vi "TestExec.Data to RetDataStr.vi"(3 "error in":errorcluster, 5 "Data":variant) -> (0 "error out":errorcluster, 2 "RetStr":string)   [LabVIEW 2017]
uses:
  <vilib>/Utility/Data Type/NI_Data Type.lvlib
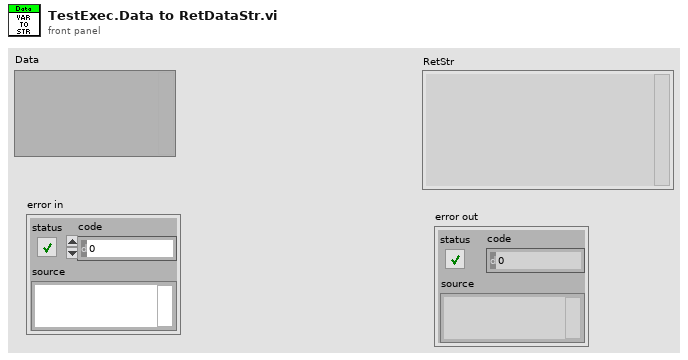
[diagram p1: front panel]
types:
  T1 = typedef "NI_Data Type.lvlib/Data Type.ctl" = enum8{"Invalid Type", "Void", "I8", "I16", "I32", "I64", "U8", "U16", "U32", "U64", "Single Float", "Double Float", "Extended Float", "Single Complex", "Double Complex", "Extended Complex", "Enum U8", "Enum U16", "Enum U32", "Enum U64", "Single Float With Unit", "Double Float With Unit", "Extended Float With Unit", "Single Complex with Unit", "Double Complex with Unit", "Extended Complex with Unit", "Boolean", "String", "Path", "Picture", "Tag", "Array", "Cluster", "Variant", "LV Variant", "Waveform", "Timestamp", "Digital Waveform", "Digital Data", "ExpressData", "Refnum", "External Data", "VI", "Poly VI", "LabVIEW Class Instance", "Fixed Point"}
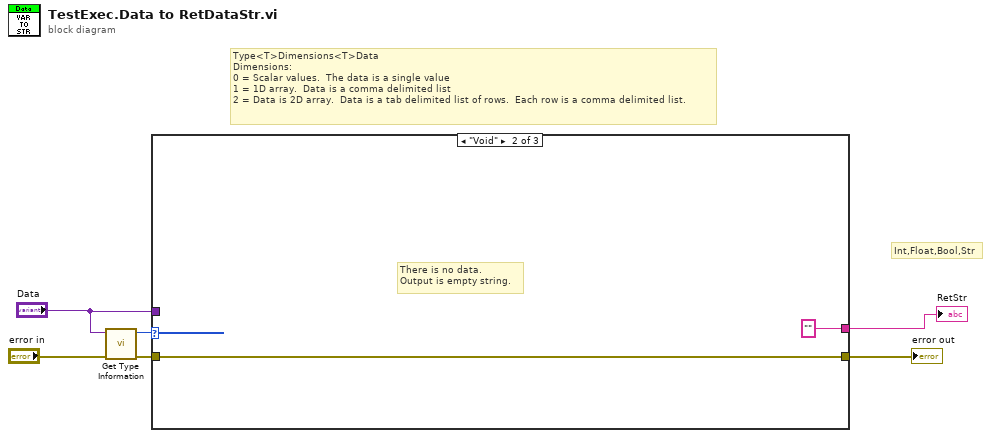
[diagram p0: block diagram]
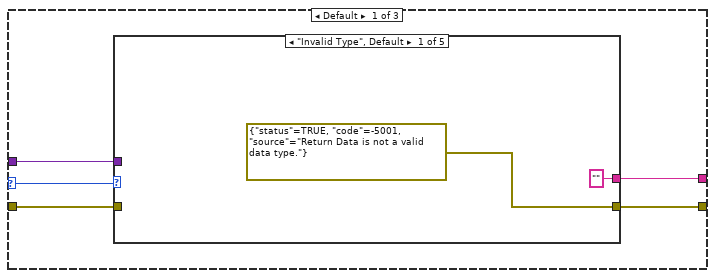
[diagram p2: hidden frame]
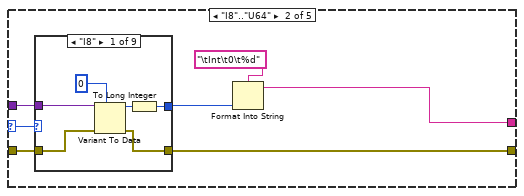
[diagram p3: hidden frame]
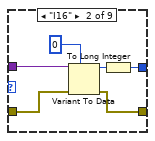
[diagram p4: hidden frame]
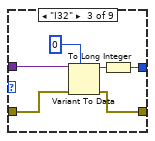
[diagram p5: hidden frame]
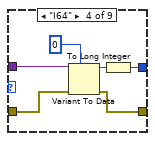
[diagram p6: hidden frame]
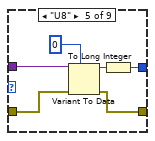
[diagram p7: hidden frame]
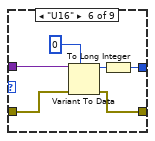
[diagram p8: hidden frame]
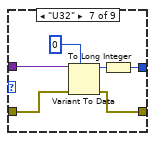
[diagram p9: hidden frame]
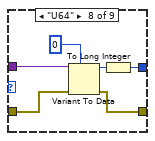
[diagram p10: hidden frame]
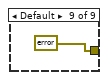
[diagram p11: hidden frame]
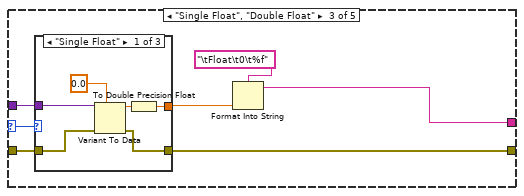
[diagram p12: hidden frame]
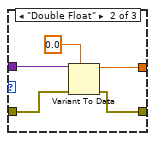
[diagram p13: hidden frame]
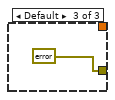
[diagram p14: hidden frame]
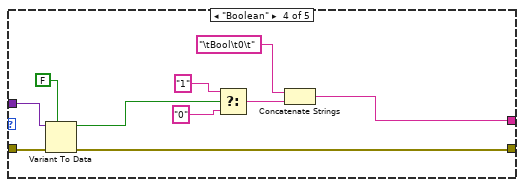
[diagram p15: hidden frame]
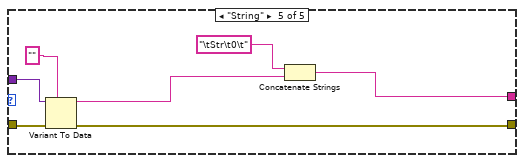
[diagram p16: hidden frame]
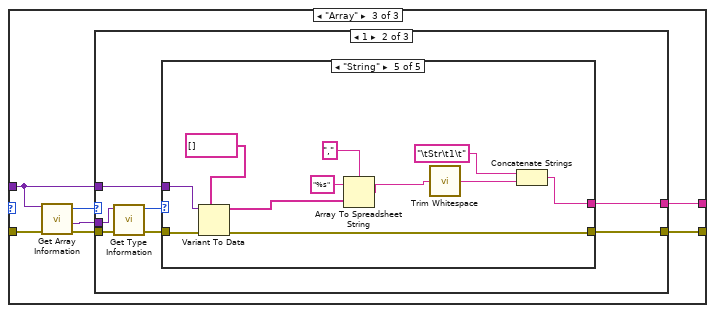
[diagram p17: hidden frame]
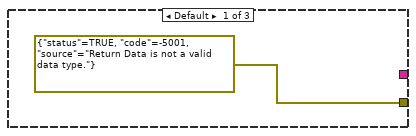
[diagram p18: hidden frame]
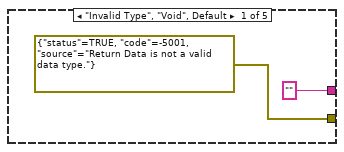
[diagram p19: hidden frame]
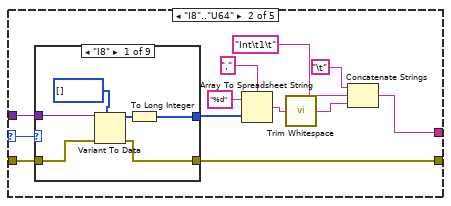
[diagram p20: hidden frame]
diagram:
  # "Type<T>Dimensions<T>Data\nDimensions:\n0 = Scalar values.  The data is a single value\n1 = 1D array.  Data is a comma delimited list\n2 = Data is 2D array.  Data is a tab delimited list of rows.  Each row is a comma delimited list."
  # "Int,Float,Bool,Str"
  n1 = call <vilib>:"Get Type Information.vi"("error in (no error)"="error in", "Variant"="Data") -> ("error out"=w5:errorcluster, "Type"=w3:T1)  [unwired: 5 in, 3 out]
  n2 = case shown="\"Void\"" w3 {
    selector: w3 -> [w7 _ _]
    tunnel: w5 -> [w11 w106 w112]
    tunnel: "Data" -> [w10 _ w111]
    tunnel: [w9 "" w114] -> w1
    tunnel: [w8 w106 w113] -> w4
    frame Default {
      n3 = case shown="\"Invalid Type\", Default" w7 {
        selector: w7 -> [_ w19 w75 _ _]
        tunnel: w11 -> [_ w18 w74 w98 w105]
        tunnel: [errorcluster {"status"=TRUE, "code"=-5001, "source"="Return Data is not a valid data type."} ("error constant") w15 w71 w89 w101] -> w8
        tunnel: ["" w16 w72 w90 w102] -> w9
        tunnel: w10 -> [_ w20 w76 w97 w104]
        frame "Invalid Type", Default {
        }
        frame "I8".."U64" {
          n4 = case shown="\"I8\"" w19 {
            tunnel: w20 -> [w26 w32 w38 w44 w50 w56 w62 w68 _]
            tunnel: [w23 w29 w35 w41 w47 w53 w59 w65 _] -> w17
            tunnel: w18 -> [w22 w28 w34 w40 w46 w52 w58 w64 _]
            tunnel: [w21 w27 w33 w39 w45 w51 w57 w63 errorcluster {"status"=TRUE, "code"=-5001, "source"="Return Data is not a valid data type."} ("error constant")] -> w15
            frame "I8" {
              n5 = Variant To Data(error in=w22, type=i8 0, Variant=w26) -> (data=w24:i8, error out=w21:errorcluster)
              n6 = To Long Integer(number=w24) -> (32bit integer=w23:i32)
            }
            frame "I16" {
              n7 = Variant To Data(error in=w28, type=i16 0, Variant=w32) -> (data=w30:i16, error out=w27:errorcluster)
              n8 = To Long Integer(number=w30) -> (32bit integer=w29:i32)
            }
            frame "I32" {
              n9 = Variant To Data(error in=w34, type=0, Variant=w38) -> (data=w36:i32, error out=w33:errorcluster)
              n10 = To Long Integer(number=w36) -> (32bit integer=w35:i32)
            }
            frame "I64" {
              n11 = Variant To Data(error in=w40, type=i64 0, Variant=w44) -> (data=w42:i64, error out=w39:errorcluster)
              n12 = To Long Integer(number=w42) -> (32bit integer=w41:i32)
            }
            frame "U8" {
              n13 = Variant To Data(error in=w46, type=u8 0, Variant=w50) -> (data=w48:u8, error out=w45:errorcluster)
              n14 = To Long Integer(number=w48) -> (32bit integer=w47:i32)
            }
            frame "U16" {
              n15 = Variant To Data(error in=w52, type=u16 0, Variant=w56) -> (data=w54:u16, error out=w51:errorcluster)
              n16 = To Long Integer(number=w54) -> (32bit integer=w53:i32)
            }
            frame "U32" {
              n17 = Variant To Data(error in=w58, type=u32 0, Variant=w62) -> (data=w60:u32, error out=w57:errorcluster)
              n18 = To Long Integer(number=w60) -> (32bit integer=w59:i32)
            }
            frame "U64" {
              n19 = Variant To Data(error in=w64, type=u64 0, Variant=w68) -> (data=w66:u64, error out=w63:errorcluster)
              n20 = To Long Integer(number=w66) -> (32bit integer=w65:i32)
            }
            frame Default {
            }
          }
          n21 = Format Into String(format string="\tInt\t0\t%d", w17) -> (resulting string=w16:string)  [unwired: 2 in, 1 out]
        }
        frame "Single Float", "Double Float" {
          n22 = case shown="\"Single Float\"" w75 {
            tunnel: w76 -> [w82 w87 _]
            tunnel: [w79 w83 _] -> w73
            tunnel: w74 -> [w78 w85 _]
            tunnel: [w77 w84 errorcluster {"status"=TRUE, "code"=-5001, "source"="Return Data is not a valid data type."} ("error constant")] -> w71
            frame "Single Float" {
              n23 = Variant To Data(error in=w78, type=sgl 0.0, Variant=w82) -> (data=w80:sgl, error out=w77:errorcluster)
              n24 = To Double Precision Float(number=w80) -> (double precision float=w79:dbl)
            }
            frame "Double Float" {
              n25 = Variant To Data(error in=w85, type=0.0, Variant=w87) -> (data=w83:dbl, error out=w84:errorcluster)
            }
            frame Default {
            }
          }
          n26 = Format Into String(format string="\tFloat\t0\t%f", w73) -> (resulting string=w72:string)  [unwired: 2 in, 1 out]
        }
        frame "Boolean" {
          n27 = Variant To Data(error in=w98, type=FALSE, Variant=w97) -> (data=w95:bool, error out=w89:errorcluster)
          n28 = Select(t="1", s=w95, f="0") -> (s? t:f=w94:string)
          n29 = Concatenate Strings("\tBool\t0\t", w94) -> (w90:string)
        }
        frame "String" {
          n30 = Variant To Data(error in=w105, type="", Variant=w104) -> (data=w99:string, error out=w101:errorcluster)
          n31 = Concatenate Strings("\tStr\t0\t", w99) -> (w102:string)
        }
      }
    }
    frame "Void" {
      # "There is no data.\nOutput is empty string."
    }
    frame "Array" {
      n32 = call <vilib>:"Get Array Information.vi"("error in (no error)"=w112, "Variant"=w111) -> ("error out"=w110:errorcluster, "Array Element Data Type"=w108:variant, "Number of Dimensions"=w109:i32)  [unwired: 6 in, 1 out]
      n33 = case shown="1" w109 {
        tunnel: [_ w122 w239] -> w114
        tunnel: [errorcluster {"status"=TRUE, "code"=-5001, "source"="Return Data is not a valid data type."} ("error constant") w121 w238] -> w113
        tunnel: w111 -> [_ w120 w237]
        tunnel: w110 -> [_ w119 w236]
        tunnel: w108 -> [_ w118 w235]
        frame Default {
        }
        frame 1 {
          n34 = call <vilib>:"Get Type Information.vi"("error in (no error)"=w119, "Variant"=w118) -> ("error out"=w116:errorcluster, "Type"=w117:T1)  [unwired: 5 in, 3 out]
          n35 = case shown="\"String\"" w117 {
            selector: w117 -> [_ w135 w195 _ _]
            tunnel: w116 -> [_ w134 w194 w221 w232]
            tunnel: [errorcluster {"status"=TRUE, "code"=-5001, "source"="Return Data is not a valid data type."} ("error constant") w133 w193 w217 w228] -> w121
            tunnel: ["" w128 w188 w218 w229] -> w122
            tunnel: w120 -> [_ w136 w196 w220 w231]
            frame "Invalid Type", "Void", Default {
            }
            frame "I8".."U64" {
              n36 = case shown="\"I8\"" w135 {
                tunnel: w136 -> [w142 w148 w153 w159 w165 w171 w177 w183 _]
                tunnel: [w140 w146 w149 w157 w163 w169 w175 w181 _] -> w132
                tunnel: w134 -> [w139 w145 w152 w156 w162 w168 w174 w180 _]
                tunnel: [w138 w144 w151 w155 w161 w167 w173 w179 errorcluster {"status"=TRUE, "code"=-5001, "source"="Return Data is not a valid data type."} ("error constant")] -> w133
                frame "I8" {
                  n37 = Variant To Data(error in=w139, type=i8[] [], Variant=w142) -> (data=w141:i8[], error out=w138:errorcluster)
                  n38 = To Long Integer(number=w141) -> (32bit integer=w140:i32[])
                }
                frame "I16" {
                  n39 = Variant To Data(error in=w145, type=i16[] [], Variant=w148) -> (data=w147:i16[], error out=w144:errorcluster)
                  n40 = To Long Integer(number=w147) -> (32bit integer=w146:i32[])
                }
                frame "I32" {
                  n41 = Variant To Data(error in=w152, type=i32[] [], Variant=w153) -> (data=w149:i32[], error out=w151:errorcluster)
                }
                frame "I64" {
                  n42 = Variant To Data(error in=w156, type=i64[] [], Variant=w159) -> (data=w158:i64[], error out=w155:errorcluster)
                  n43 = To Long Integer(number=w158) -> (32bit integer=w157:i32[])
                }
                frame "U8" {
                  n44 = Variant To Data(error in=w162, type=u8[] [], Variant=w165) -> (data=w164:u8[], error out=w161:errorcluster)
                  n45 = To Long Integer(number=w164) -> (32bit integer=w163:i32[])
                }
                frame "U16" {
                  n46 = Variant To Data(error in=w168, type=u16[] [], Variant=w171) -> (data=w170:u16[], error out=w167:errorcluster)
                  n47 = To Long Integer(number=w170) -> (32bit integer=w169:i32[])
                }
                frame "U32" {
                  n48 = Variant To Data(error in=w174, type=u32[] [], Variant=w177) -> (data=w176:u32[], error out=w173:errorcluster)
                  n49 = To Long Integer(number=w176) -> (32bit integer=w175:i32[])
                }
                frame "U64" {
                  n50 = Variant To Data(error in=w180, type=u64[] [], Variant=w183) -> (data=w182:u64[], error out=w179:errorcluster)
                  n51 = To Long Integer(number=w182) -> (32bit integer=w181:i32[])
                }
                frame Default {
                }
              }
              n52 = Array To Spreadsheet String(delimiter (Tab)=",", array=w132, 3:"%d" ("format string")) -> (spreadsheet string=w127:string)
              n53 = call <vilib>:"Trim Whitespace.vi"("string"=w127) -> ("trimmed string"=w126:string)  [unwired: 1 in]
              n54 = Concatenate Strings("\t", "Int\t1\t", w126) -> (w128:string)
            }
            frame "Single Float", "Double Float" {
              n55 = case shown="\"Single Float\"" w195 {
                tunnel: w196 -> [w202 w207 _]
                tunnel: [w200 w204 _] -> w190
                tunnel: w194 -> [w199 w206 _]
                tunnel: [w198 w205 errorcluster {"status"=TRUE, "code"=-5001, "source"="Return Data is not a valid data type."} ("error constant")] -> w193
                frame "Single Float" {
                  n56 = Variant To Data(error in=w199, type=sgl[] [], Variant=w202) -> (data=w201:sgl[], error out=w198:errorcluster)
                  n57 = To Double Precision Float(number=w201) -> (double precision float=w200:dbl[])
                }
                frame "Double Float" {
                  n58 = Variant To Data(error in=w206, type=dbl[] [], Variant=w207) -> (data=w204:dbl[], error out=w205:errorcluster)
                }
                frame Default {
                }
              }
              n59 = Array To Spreadsheet String(delimiter (Tab)=",", array=w190, 3:"%f" ("format string")) -> (spreadsheet string=w187:string)
              n60 = call <vilib>:"Trim Whitespace.vi"("string"=w187) -> ("trimmed string"=w186:string)  [unwired: 1 in]
              n61 = Concatenate Strings("\t", "Float\t1\t", w186) -> (w188:string)
            }
            frame "Boolean" {
              n62 = Variant To Data(error in=w221, type=bool[] [], Variant=w220) -> (data=w215:bool[], error out=w217:errorcluster)
              n63 = Boolean To (0,1)(Boolean=w215) -> (0, 1=w212:i16[])
              n64 = Array To Spreadsheet String(delimiter (Tab)=",", array=w212, 3:"%d" ("format string")) -> (spreadsheet string=w211:string)
              n65 = call <vilib>:"Trim Whitespace.vi"("string"=w211) -> ("trimmed string"=w210:string)  [unwired: 1 in]
              n66 = Concatenate Strings("\t", "Bool\t1\t", w210) -> (w218:string)
            }
            frame "String" {
              n67 = Variant To Data(error in=w232, type=string[] [], Variant=w231) -> (data=w224:string[], error out=w228:errorcluster)
              n68 = Array To Spreadsheet String(delimiter (Tab)=",", array=w224, 3:"%s" ("format string")) -> (spreadsheet string=w223:string)
              n69 = call <vilib>:"Trim Whitespace.vi"("string"=w223) -> ("trimmed string"=w222:string)  [unwired: 1 in]
              n70 = Concatenate Strings("\tStr\t1\t", w222) -> (w229:string)
            }
          }
        }
        frame 2 {
          n71 = call <vilib>:"Get Type Information.vi"("error in (no error)"=w236, "Variant"=w235) -> ("error out"=w233:errorcluster, "Type"=w234:T1)  [unwired: 5 in, 3 out]
          n72 = case shown="\"I8\"..\"U64\"" w234 {
            selector: w234 -> [_ w255 w318 _ _]
            tunnel: w233 -> [_ w254 w317 w347 w362]
            tunnel: [errorcluster {"status"=TRUE, "code"=-5001, "source"="Return Data is not a valid data type."} ("error constant") w253 w316 w343 w358] -> w238
            tunnel: ["" w248 w311 w344 w359] -> w239
            tunnel: w237 -> [_ w256 w319 w346 w361]
            frame "Invalid Type", "Void", Default {
            }
            frame "I8".."U64" {
              n73 = case shown="\"I32\"" w255 {
                tunnel: w256 -> [w262 w268 w273 w279 w285 w291 w297 _ w304]
                tunnel: [w260 w266 w269 w277 w283 w289 w295 _ w302] -> w252
                tunnel: w254 -> [w259 w265 w272 w276 w282 w288 w294 _ w301]
                tunnel: [w258 w264 w271 w275 w281 w287 w293 errorcluster {"status"=TRUE, "code"=-5001, "source"="Return Data is not a valid data type."} ("error constant") w300] -> w253
                frame "I8" {
                  n74 = Variant To Data(error in=w259, type=i8[][] [], Variant=w262) -> (data=w261:i8[][], error out=w258:errorcluster)
                  n75 = To Long Integer(number=w261) -> (32bit integer=w260:i32[][])
                }
                frame "I16" {
                  n76 = Variant To Data(error in=w265, type=i16[][] [], Variant=w268) -> (data=w267:i16[][], error out=w264:errorcluster)
                  n77 = To Long Integer(number=w267) -> (32bit integer=w266:i32[][])
                }
                frame "I32" {
                  n78 = Variant To Data(error in=w272, type=i32[][] [], Variant=w273) -> (data=w269:i32[][], error out=w271:errorcluster)
                }
                frame "I64" {
                  n79 = Variant To Data(error in=w276, type=i64[][] [], Variant=w279) -> (data=w278:i64[][], error out=w275:errorcluster)
                  n80 = To Long Integer(number=w278) -> (32bit integer=w277:i32[][])
                }
                frame "U8" {
                  n81 = Variant To Data(error in=w282, type=u8[][] [], Variant=w285) -> (data=w284:u8[][], error out=w281:errorcluster)
                  n82 = To Long Integer(number=w284) -> (32bit integer=w283:i32[][])
                }
                frame "U16" {
                  n83 = Variant To Data(error in=w288, type=u16[][] [], Variant=w291) -> (data=w290:u16[][], error out=w287:errorcluster)
                  n84 = To Long Integer(number=w290) -> (32bit integer=w289:i32[][])
                }
                frame "U32" {
                  n85 = Variant To Data(error in=w294, type=u32[][] [], Variant=w297) -> (data=w296:u32[][], error out=w293:errorcluster)
                  n86 = To Long Integer(number=w296) -> (32bit integer=w295:i32[][])
                }
                frame Default {
                }
                frame "U64" {
                  n87 = Variant To Data(error in=w301, type=u64[][] [], Variant=w304) -> (data=w303:u64[][], error out=w300:errorcluster)
                  n88 = To Long Integer(number=w303) -> (32bit integer=w302:i32[][])
                }
              }
              n89 = Array To Spreadsheet String(delimiter (Tab)=",", array=w252, 3:"%d" ("format string")) -> (spreadsheet string=w243:string)
              n90 = call <vilib>:"Trim Whitespace.vi"("string"=w243) -> ("trimmed string"=w247:string)  [unwired: 1 in]
              n91 = call <vilib>:"Search and Replace Pattern.vi"("string"=w247, "regular expression (\"\")"="\r\n", "replace string (\"\")"="\t", "replace all? (F)"=TRUE) -> ("result string"=w242:string)  [unwired: 1 in, 1 out]
              n92 = Concatenate Strings("\tInt\t2\t", w242) -> (w248:string)
            }
            frame "Single Float", "Double Float" {
              n93 = case shown="Default" w318 {
                tunnel: w319 -> [w325 w330 _]
                tunnel: [w323 w327 _] -> w313
                tunnel: w317 -> [w322 w329 _]
                tunnel: [w321 w328 errorcluster {"status"=TRUE, "code"=-5001, "source"="Return Data is not a valid data type."} ("error constant")] -> w316
                frame "Single Float" {
                  n94 = Variant To Data(error in=w322, type=sgl[][] [], Variant=w325) -> (data=w324:sgl[][], error out=w321:errorcluster)
                  n95 = To Double Precision Float(number=w324) -> (double precision float=w323:dbl[][])
                }
                frame "Double Float" {
                  n96 = Variant To Data(error in=w329, type=dbl[][] [], Variant=w330) -> (data=w327:dbl[][], error out=w328:errorcluster)
                }
                frame Default {
                }
              }
              n97 = Array To Spreadsheet String(delimiter (Tab)=",", array=w313, 3:"%f" ("format string")) -> (spreadsheet string=w306:string)
              n98 = call <vilib>:"Trim Whitespace.vi"("string"=w306) -> ("trimmed string"=w310:string)  [unwired: 1 in]
              n99 = call <vilib>:"Search and Replace Pattern.vi"("string"=w310, "regular expression (\"\")"="\r\n", "replace string (\"\")"="\t", "replace all? (F)"=TRUE) -> ("result string"=w305:string)  [unwired: 1 in, 1 out]
              n100 = Concatenate Strings("\tFloat\t2\t", w305) -> (w311:string)
            }
            frame "Boolean" {
              n101 = Variant To Data(error in=w347, type=bool[][] [], Variant=w346) -> (data=w341:bool[][], error out=w343:errorcluster)
              n102 = Boolean To (0,1)(Boolean=w341) -> (0, 1=w338:i16[][])
              n103 = Array To Spreadsheet String(delimiter (Tab)=",", array=w338, 3:"%d" ("format string")) -> (spreadsheet string=w334:string)
              n104 = call <vilib>:"Trim Whitespace.vi"("string"=w334) -> ("trimmed string"=w337:string)  [unwired: 1 in]
              n105 = call <vilib>:"Search and Replace Pattern.vi"("string"=w337, "regular expression (\"\")"="\r\n", "replace string (\"\")"="\t", "replace all? (F)"=TRUE) -> ("result string"=w333:string)  [unwired: 1 in, 1 out]
              n106 = Concatenate Strings("\tBool\t2\t", w333) -> (w344:string)
            }
            frame "String" {
              n107 = Variant To Data(error in=w362, type=string[][] [], Variant=w361) -> (data=w354:string[][], error out=w358:errorcluster)
              n108 = Array To Spreadsheet String(delimiter (Tab)=",", array=w354, 3:"%s" ("format string")) -> (spreadsheet string=w349:string)
              n109 = call <vilib>:"Trim Whitespace.vi"("string"=w349) -> ("trimmed string"=w353:string)  [unwired: 1 in]
              n110 = call <vilib>:"Search and Replace Pattern.vi"("string"=w353, "regular expression (\"\")"="\r\n", "replace string (\"\")"="\t", "replace all? (F)"=TRUE) -> ("result string"=w348:string)  [unwired: 1 in, 1 out]
              n111 = Concatenate Strings("\tStr\t2\t", w348) -> (w359:string)
            }
          }
        }
      }
    }
  }
  "RetStr" <- w1
  "error out" <- w4
